vi "Config Interface View.vi"(8 "error in (no error)":errorcluster, 11 "View Model":T1) -> (0 "error out":errorcluster, 3 "View Model":T1)   [LabVIEW 2017]
doc: "Separated UI for Config DB provides full access to the data records"
uses:
  Configuration Database/Controls/Config Commands.ctl
  Configuration Database/Controls/Congif Data.ctl
  View Model/Controls/View Model.ctl
  Configuration Database/Controls/Config Model.ctl
  View Model/Controls/Shared Model.ctl
  Error Handler/Controls/Error Model.ctl
  Error Handler/Controls/Error Data.ctl
  Error Handler/Controls/Error Type.ctl
  Car Wash Controller/Controls/Car Wash Model.ctl
  Car Wash Controller/Controls/Car Wash States.ctl
  Car Wash Controller/Controls/Controller Overhead.ctl
  Car Wash Controller/Controls/Vehicle Location.ctl
  Car Wash Controller/Controls/CarWash CMD.ctl
panel:
  in  "Config Data":T6 {"Step Duration" max=99999 step=1}
  in  "Stop":bool
  out "Configuration Data records":string
  in  "Config Command":T7
  # "[Covers: SD6]"
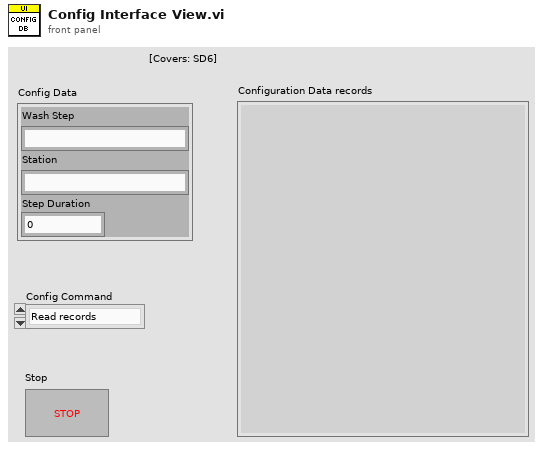
[diagram p1: front panel]
types:
  T1 = typedef "View Model.ctl" = cluster{"Config Model":T2, "Shared Model":T3, "Error Model":T4, "Car Wash Model":T5}
  T2 = typedef "Config Model.ctl" = cluster{"Config Event":refnum<user-event>, "Config DVR":refnum<data-value>, "Config CMD":refnum<user-event>, "Config Locked?":refnum<data-value>}
  T3 = typedef "Shared Model.ctl" = cluster{"Stop event":refnum<user-event>, "Stop DVR":refnum<data-value>}
  T4 = typedef "Error Model.ctl" = cluster{"Error event":refnum<user-event>, "Error DVR":refnum<data-value>}
  T5 = typedef "Car Wash Model.ctl" = cluster{"State Change":refnum<user-event>, "Out of Position Change":refnum<user-event>, "Wash Entry Change":refnum<user-event>, "Contr Overhead DVR":refnum<data-value>, "Contr Overhead Event":refnum<user-event>, "CarWash CMD":refnum<user-event>, "Location Change":refnum<user-event>}
  T6 = typedef "Congif Data.ctl" = cluster{"Wash Step":string, "Station":string, "Step Duration":u32}
  T7 = typedef "Config Commands.ctl" = enum16{"Read records", "Query timing data", "Insert new data records", "Update data records"}
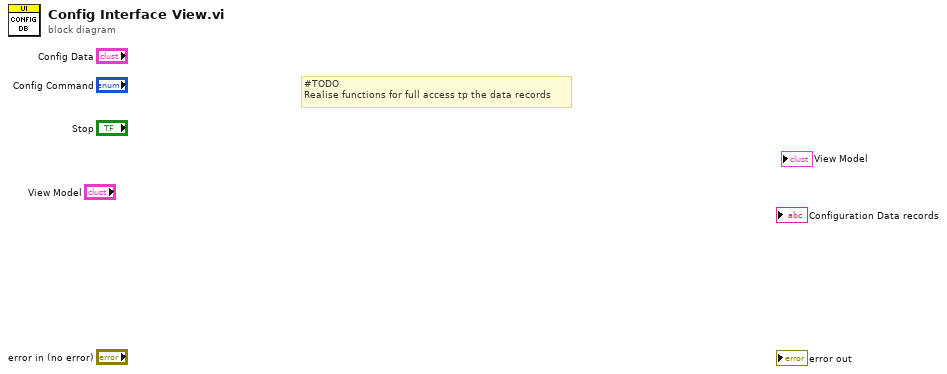
[diagram p0: block diagram]
diagram:
  # "#TODO\nRealise functions for full access tp the data records"
